vi "Receive Message.vi"(6 "priority":i32, 10 "Driver in in":refnum<class "Driver.lvclass">, 11 "Message in":refnum<class "Message.lvclass">) -> (0 "error out":errorcluster, 2 "Actor out":refnum<class "Actor.lvclass">)   [LabVIEW 2013, in "Logical Systems.lvlib" / "Driver.lvlib" / "Driver.lvclass"]
doc: "This VI should be overriden ONLY if you are creating a proxy actor for remote transmission. If you are, override this VI to transmit the received message to a new destination, maintaining the given priority."
uses:
  Driver.lvclass
  <vilib>/ActorFramework/Message/Message.lvclass
  <vilib>/ActorFramework/Actor/Actor.lvclass
  Robot Actors/System Actor/System Actor Class/System Actor.lvclass
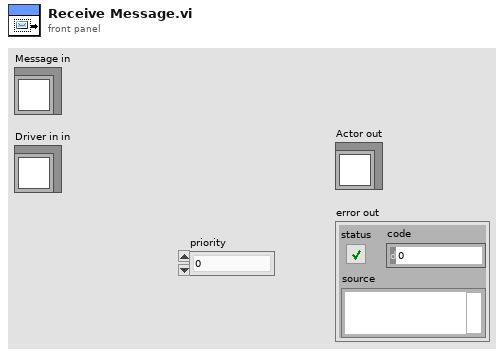
[diagram p1: front panel]
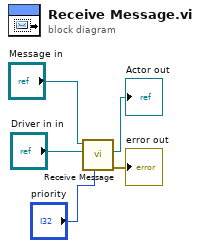
[diagram p0: block diagram]
diagram:
  n1 = call-parent "Receive Message.vi"("priority"="priority", "System Actor in in"="Driver in in", "Message in"="Message in") -> ("error out"=→"error out":errorcluster, "Actor out"=→"Actor out":refnum<class "Actor.lvclass">)  [unwired: 7 in]
